vi "PT (Main).vi"(7 "Name of Parent Panel":string="Main.vi", 9 "New Center Coords":T1={"Horizontal"=470, "Vertical"=200}, 10 "Config":variant, 11 "Main UI Message Queue":refnum<queue>) -> ()   [LabVIEW 2018, in "PT Module.lvlib"]
doc: "This Continuous Measurement sample project is based on the Queued Message Handler template.\n\nThe Event Handling Loop generates messages based on user interface actions.\n\nThe Message Handling Loop processes messages generated by the Event Handling Loop, or by other messages. There are also Acquisition and Logging message handling loop subVIs, and a chart updating loop."
uses:
  PT Module.lvlib
  support/Message Queue/Message Cluster.ctl
  <vilib>/Utility/miscctls.llb/LVPoint32TypeDef.ctl
  Controls/PT Module Config Cluster.ctl
  Tag VIs/Numeric Alarm Settings Cluster.ctl
  Tag VIs/Tag FGV Operation Enum.ctl
  support/Message Queue/Enqueue Message (Single).vi
  support/User Event - Stop/User Event - Stop.lvlib
  support/Support Library.lvlib
  support/Message Queue/Message Queue.lvlib
  Shared Variables/Dynamic Shared Variables.lvlib
  subVIs/PT Settings Dialog.vi
  support/Command Log VIs/Command Logging.lvlib
panel:
  out "Numeric":dbl format="%.1f"
  out "data string 2":string
  out "data string":string
  out "xml string":string
  in  "Settings":bool
  out "Tag Name":string
  out "Input Channel Tag Name":string
  out "Pressure":dbl caption="PSIG" format="%.1f"
  in  "Start":bool
  out "Log File path":path
  in  "Force Trigger":bool
  in  "Stop":bool
  out "Status":string
  in  "Exit":bool
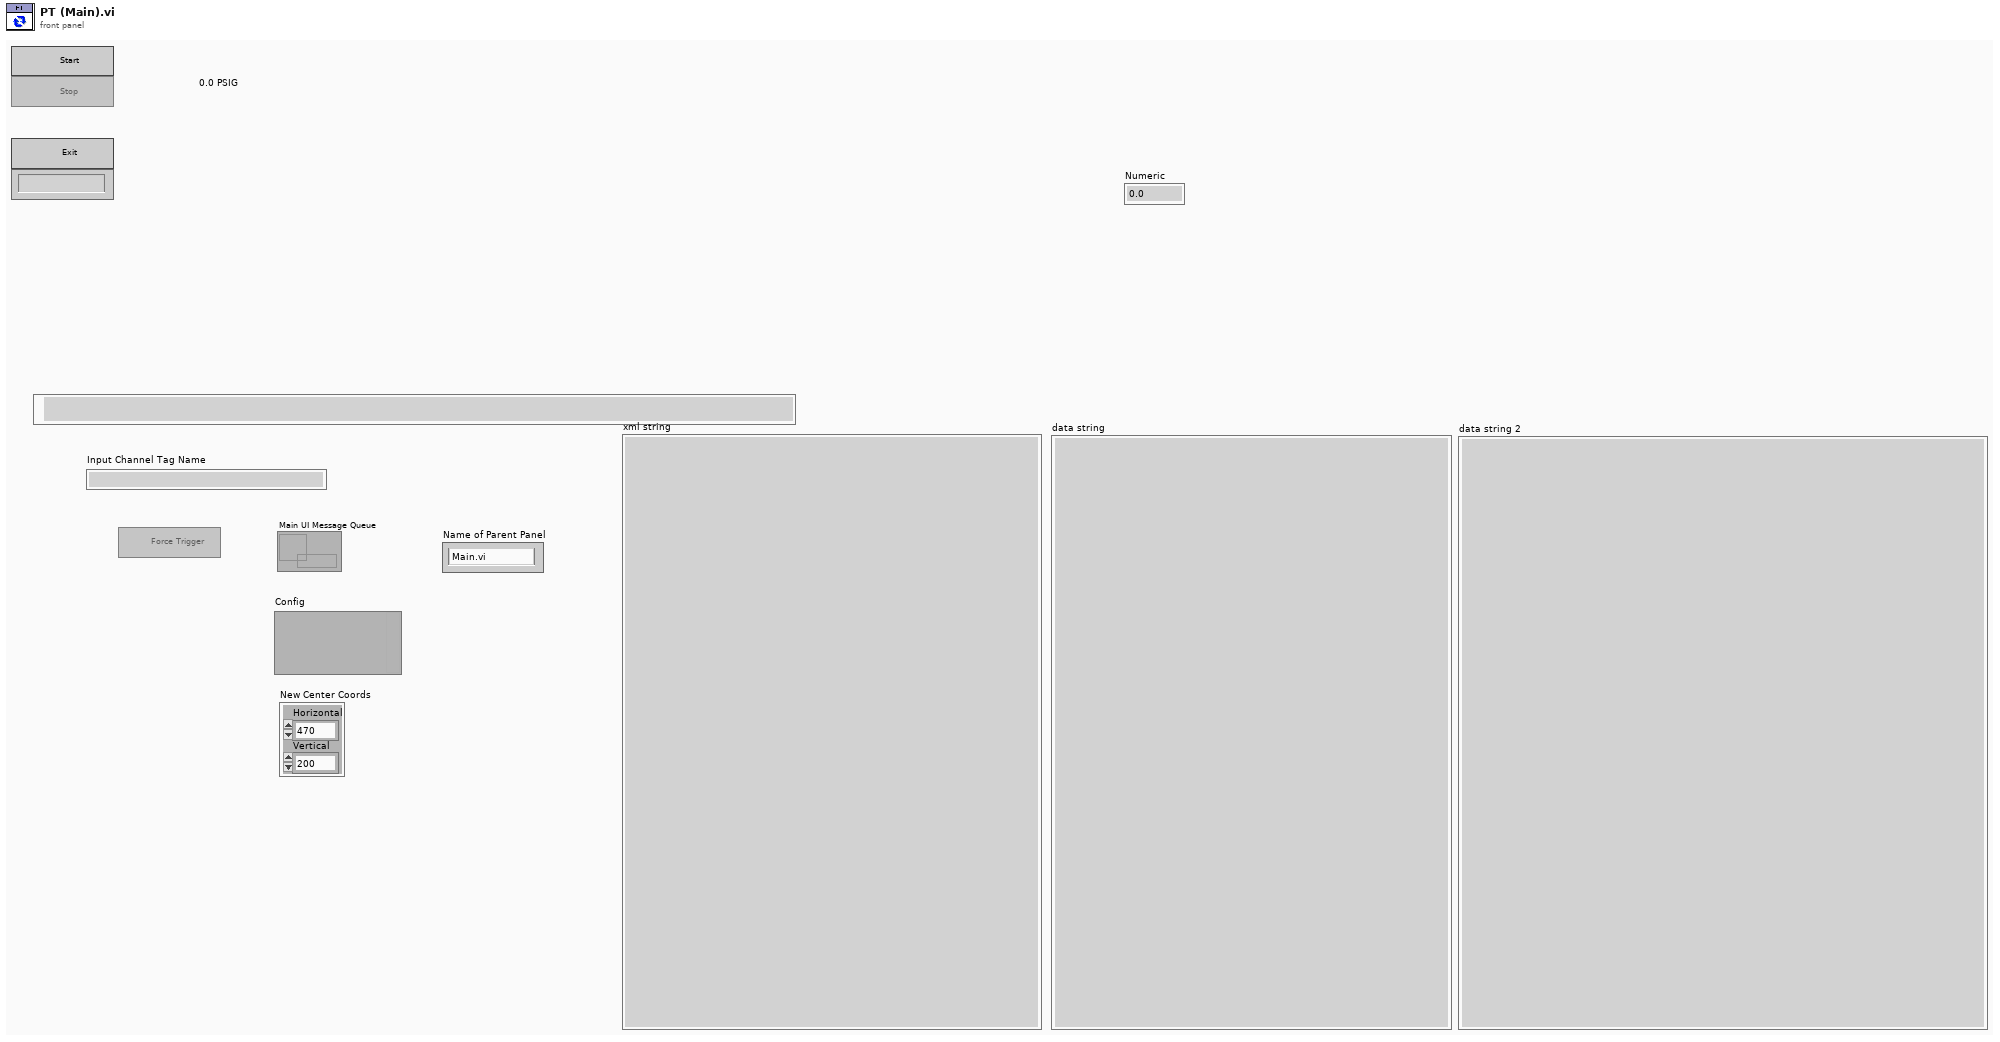
[diagram p1: front panel]
types:
  T1 = typedef "LVPoint32TypeDef.ctl" = cluster{"Horizontal":i32, "Vertical":i32}
  T2 = typedef "PT Module.lvlib/PT Module Config Cluster.ctl" = cluster{"GUID":string, "Drop Coords":T1, "Input Channel Tag Name ":string, "Process Name":string, "Queue Name":string, "Input Channel Numeric Alarm Settings":T3[]}
  T3 = typedef "Numeric Alarm Settings Cluster.ctl" = cluster{"enable? (F)":bool, "name":string, "alarm type":enum16{"HI_HI", "HI", "LO", "LO_LO"}, "level/change":dbl, "deadband/time":dbl, "alarm delay":dbl, "priority":u32, "ack type":enum16{"Auto", "User", "None", "Each Occurrence"}, "area":string, "description":string, "log? (T)":bool}
  T4 = typedef "Tag FGV Operation Enum.ctl" = enum16{"Init", "Set Notification Queue", "Create Tag", "Commit", "Write Tag (Numeric)", "Write Tag (Boolean)", "Read All Tags", "Read One Tag", "Delete Tag Category", "Set Alarm Parameters (Numeric)", "Set Alarm Parameters (Boolean)", "Enable All Alarms", "Disable All Alarms", "Delete All Tags", "Read Alarms", "Ack Alarm", "Read Alarm Parameters (Numeric)", "Read Alarm Parameters (Boolean)"}
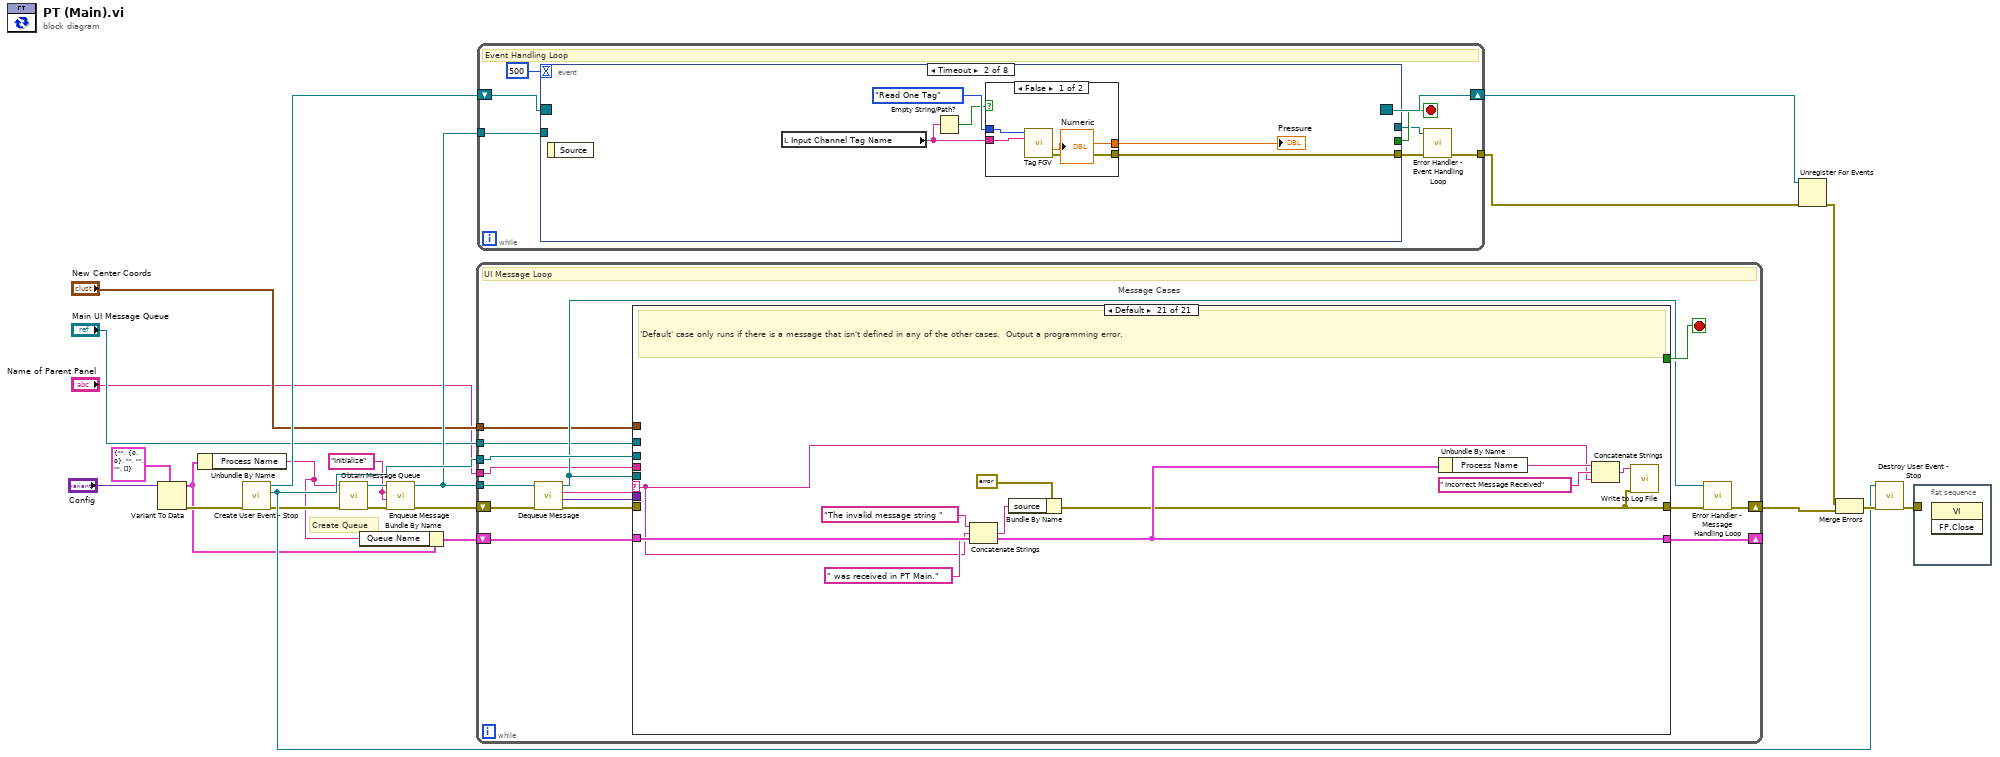
[diagram p0: block diagram]
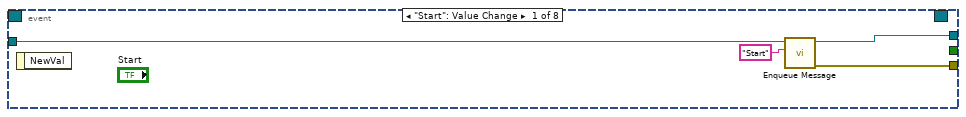
[diagram p2: hidden frame]
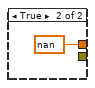
[diagram p3: hidden frame]
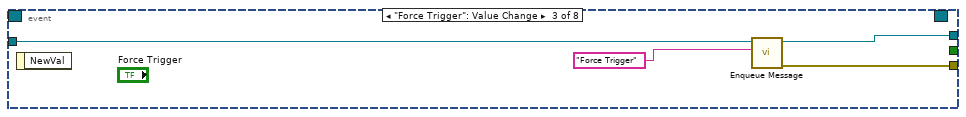
[diagram p4: hidden frame]
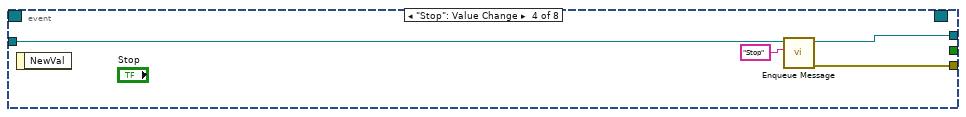
[diagram p5: hidden frame]
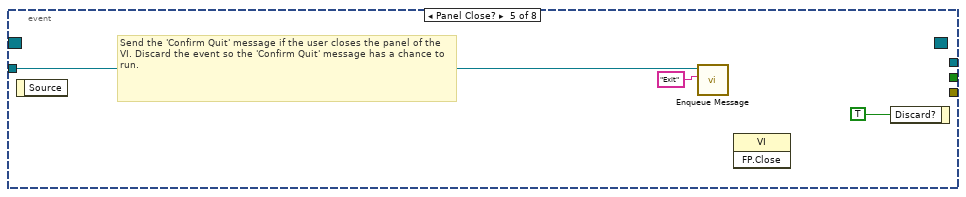
[diagram p6: hidden frame]
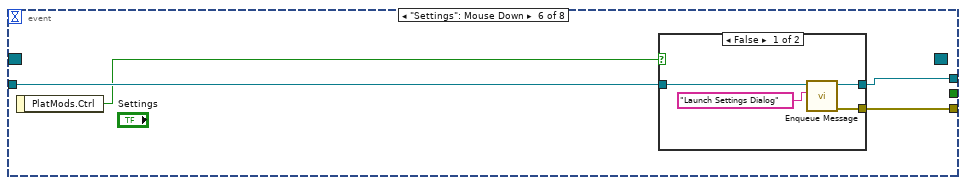
[diagram p7: hidden frame]
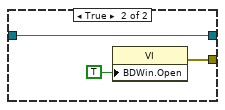
[diagram p8: hidden frame]
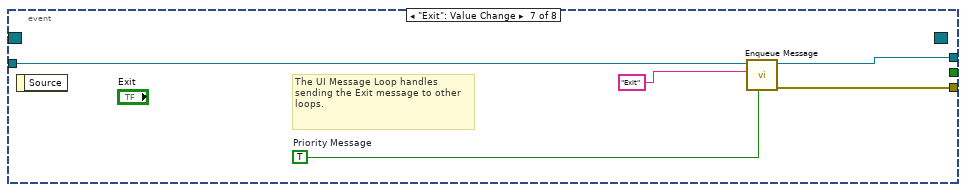
[diagram p9: hidden frame]
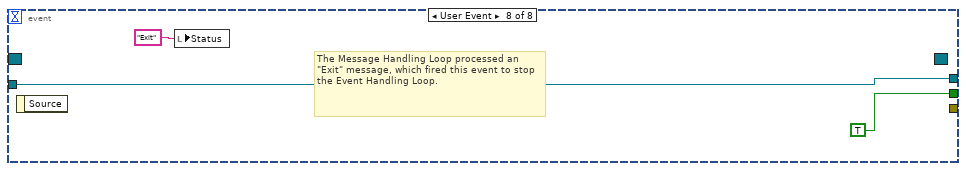
[diagram p10: hidden frame]
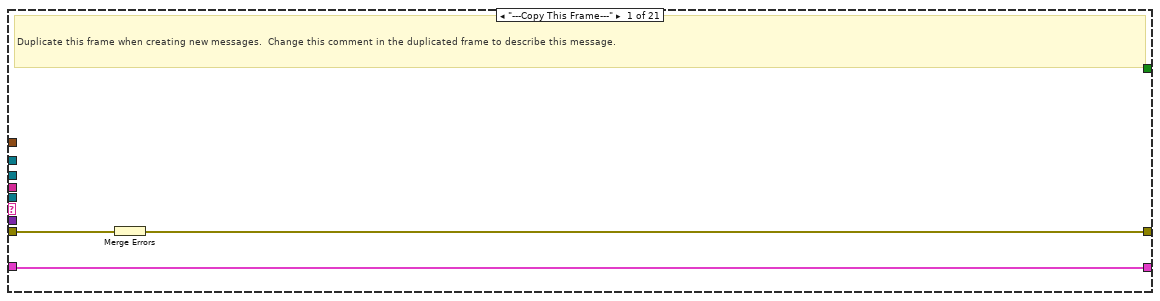
[diagram p11: hidden frame]
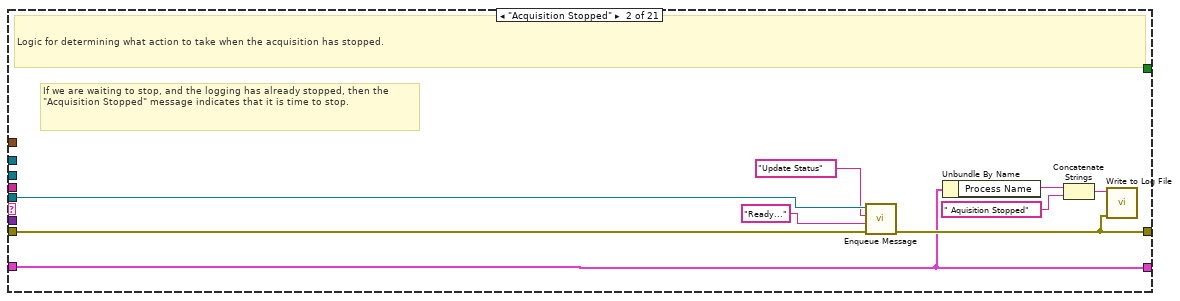
[diagram p12: hidden frame]
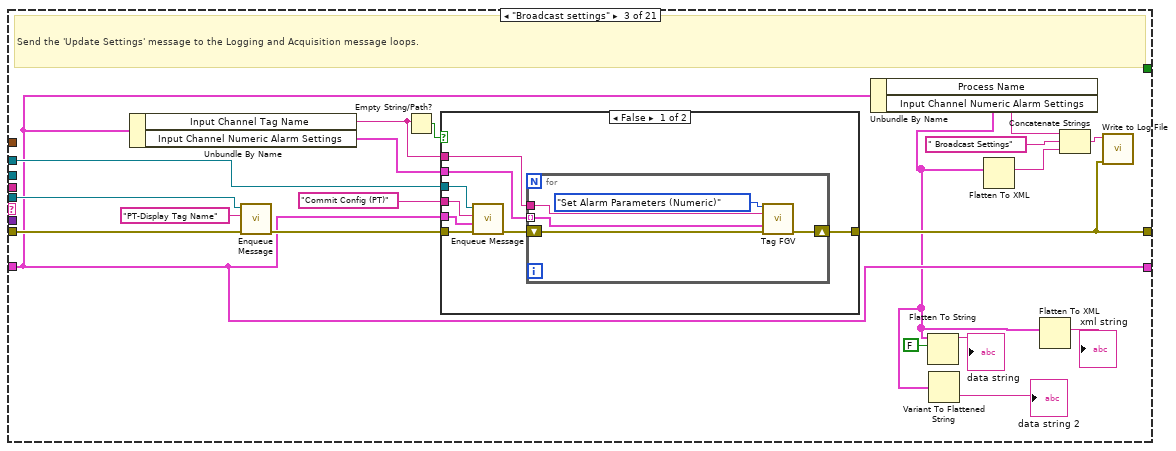
[diagram p13: hidden frame]
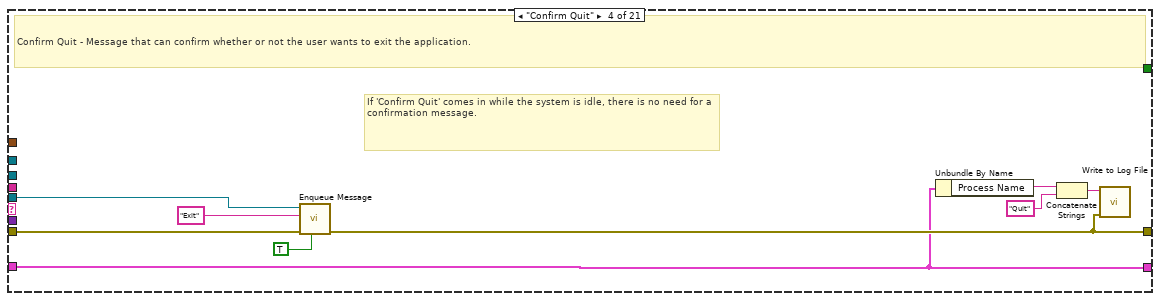
[diagram p15: hidden frame]
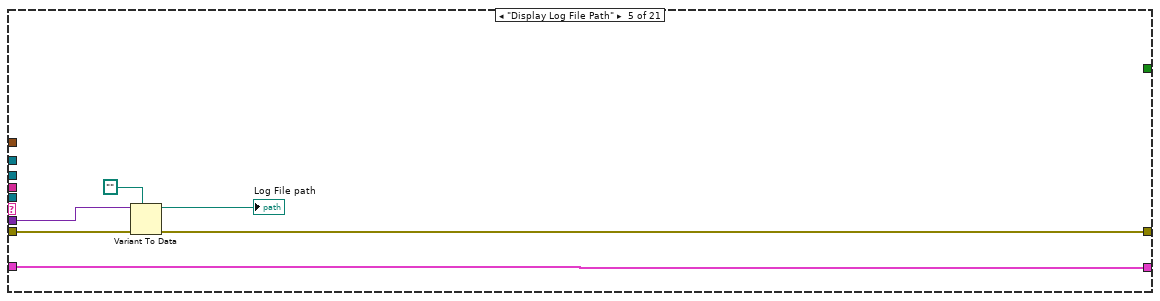
[diagram p16: hidden frame]
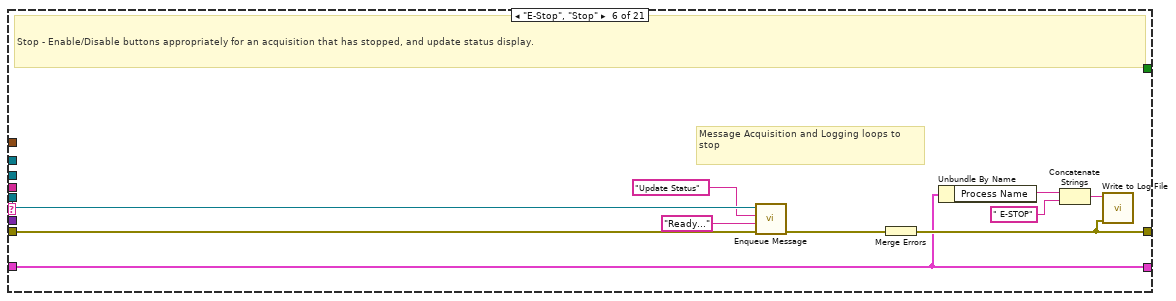
[diagram p17: hidden frame]
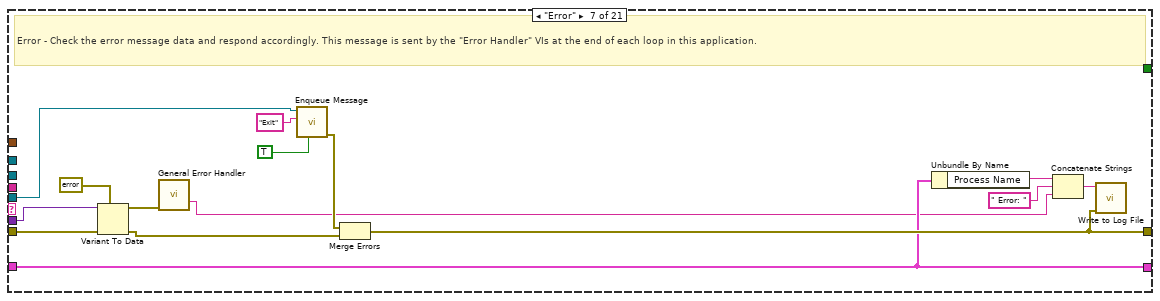
[diagram p18: hidden frame]
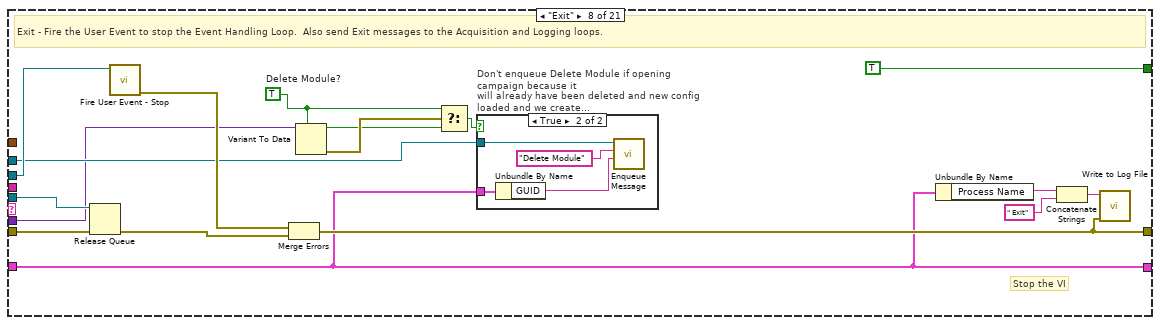
[diagram p19: hidden frame]
diagram:
  w13 = "Initialize" ("Message")
  # "Create Queue"
  n1 = Variant To Data(type=T2 {"GUID"="", "Drop Coords"={"Horizontal"=0, "Vertical"=0}, "Input Channel Tag Name "="", "Process Name"="", "Queue Name"="", "Input Channel Numeric Alarm Settings"=[]} ("TT Module Config"), Variant="Config") -> (data=w2:T2, error out=w7:errorcluster)  [unwired: 1 in]
  n2 = Unbundle By Name(w2) -> ("Process Name"=w3:string)
  n3 = call "Create User Event - Stop.vi"("error in (no error)"=w7) -> ("error out"=w11:errorcluster, "User Event - Stop"=w19:refnum<user-event>, "Stop Event Registration Refnum"=w20:refnum<event-registration>)  [unwired: 8 in]
  n4 = call "Obtain Message Queue.vi"("error in (no error)"=w11, "name (unnamed)"=w3) -> ("error out"=w16:errorcluster, "Message Queue"=w15:refnum<queue>)  [unwired: 8 in]
  n5 = Bundle By Name(cluster=w2, "Queue Name"=w3) -> (w1:T2)
  n6 = call-poly "Enqueue Message.vi"("error in (no error)"=w16, "Message Data"=w13, "Message"=w13, "Message Queue"=w15) -> ("error out"=w12:errorcluster, "dup Message Queue"=w14:refnum<queue>)  [unwired: 6 in]
  n7 = while {
    tunnel: w14 -> [w32]
    tunnel: w19 -> [w37]
    shift-right: [w28] -> w23
    shift-left: w12 -> [w36]
    shift-right: [w31] -> _
    shift-left: w1 -> [w30]
    tunnel: "Main UI Message Queue" -> [w26]
    tunnel: "New Center Coords" -> [w25]
    tunnel: "Name of Parent Panel" -> [w24]
    stop <- w38 stop-if-true
    # "UI Message Loop"
    n8 = call "Dequeue Message.vi"("error in (no error)"=w36, "Message Queue"=w32) -> ("error out"=w35:errorcluster, "Message Data"=w33:variant, "Message"=w34:string, "dup Message Queue"=w27:refnum<queue>)  [unwired: 6 in]
    n9 = case "Message Cases" shown="Default" w34 {
      selector: w34 -> [_ _ _ _ _ _ _ _ _ _ _ _ _ _ _ _ _ _ _ _ w248]
      tunnel: w27 -> [_ w49 w68 w93 _ w109 w120 w137 _ _ w174 w184 _ _ w201 w206 w225 _ _ _ _]
      tunnel: w35 -> [w41 w50 w70 w92 w94 w106 w124 w140 w146 w159 w171 w188 w194 w196 w200 w207 w223 w230 w237 w245 _]
      tunnel: [w40 w43 w58 w86 w95 w101 w112 w126 w148 w159 w160 w180 w194 w196 w199 w205 w219 w230 w236 w246 w247] -> w29
      tunnel: [_ _ _ _ _ _ _ TRUE _ _ _ _ _ _ _ _ _ _ _ _ _] -> w38
      tunnel: w33 -> [_ _ _ _ w97 _ w123 w130 _ _ _ _ _ _ _ _ _ _ _ w244 _]
      tunnel: w37 -> [_ _ _ _ _ _ _ w139 _ _ _ _ _ _ _ _ _ _ _ _ _]
      tunnel: [w39 w42 w57 w85 w99 w100 w111 w125 w147 w158 w161 w179 w195 w197 w204 w210 w218 w231 w232 w241 w253] -> w31
      tunnel: w30 -> [w39 w42 w57 w85 w99 w100 w111 w125 w147 w158 w161 w185 w195 w197 w204 w210 w218 w231 w232 w241 w253]
      tunnel: w26 -> [_ _ w69 _ _ _ _ w131 _ _ _ _ _ _ _ _ _ _ w238 _ _]
      tunnel: w25 -> [_ _ _ _ _ _ _ _ _ _ w167 _ _ _ _ _ _ _ _ _ _]
      tunnel: w24 -> [_ _ _ _ _ _ _ _ _ _ w166 _ _ _ _ _ _ _ _ _ _]
      frame "---Copy This Frame---" {
        # "Duplicate this frame when creating new messages.  Change this comment in the duplicated frame to describe this message."
        n10 = Merge Errors(w41) -> (w40:errorcluster)
      }
      frame "Acquisition Stopped" {
        # "If we are waiting to stop, and the logging has already stopped, then the \"Acquisition Stopped\" message indicates that it is time to stop."
        # "Logic for determining what action to take when the acquisition has stopped."
        n11 = call-poly "Enqueue Message.vi"("error in (no error)"=w50, "Message Data"="Ready..." ("Message"), "Message"="Update Status", "Message Queue"=w49) -> ("error out"=w43:errorcluster)  [unwired: 6 in, 1 out]
        n12 = Unbundle By Name(w42) -> ("Process Name"=w46:string)
        n13 = Concatenate Strings(w46, " Aquisition Stopped" ("text")) -> (w45:string)
        n14 = call "Write to Log File.vi"("error in"=w43, "text"=w45) -> ()  [unwired: 9 in, 1 out]
      }
      frame "Broadcast settings" {
        # "Send the 'Update Settings' message to the Logging and Acquisition message loops."
        n15 = Unbundle By Name(w57) -> ("Input Channel Tag Name"=w62:string, "Input Channel Numeric Alarm Settings"=w66:T3[])
        n16 = call-poly "Enqueue Message.vi"("error in (no error)"=w70, "Message"="PT-Display Tag Name", "Message Queue"=w68) -> ("error out"=w64:errorcluster)  [unwired: 7 in, 1 out]
        n17 = Empty String/Path?(string/path=w62) -> (empty?=w65:bool)
        n18 = case shown="False" w65 {
          tunnel: w66 -> [w78 _]
          tunnel: [w77 w84] -> w58
          tunnel: w64 -> [w76 w84]
          tunnel: w57 -> [w75 _]
          tunnel: "Commit Config (PT)" ("Message") -> [w74 _]
          tunnel: w69 -> [w73 _]
          tunnel: w62 -> [w71 _]
          frame False {
            n19 = call-poly "Enqueue Message.vi"("error in (no error)"=w76, "Message Data"=w75, "Message"=w74, "Message Queue"=w73) -> ("error out"=w72:errorcluster)  [unwired: 6 in, 1 out]
            n20 = for {
              tunnel: w78 -> [w82] mode=indexing
              tunnel: w71 -> [w81]
              shift-right: [w79] -> w77
              shift-left: w72 -> [w80]
              n21 = call "Tag FGV.vi"("Operation"=Tag_FGV_Operation_Enum."Set Alarm Parameters (Numeric)", "Tag Name"=w81, "Data"=w82, "error in (no error)"=w80) -> ("error out"=w79:errorcluster)  [unwired: 4 in, 7 out]
            }
          }
          frame True {
          }
        }
        n22 = Unbundle By Name(w57) -> ("Process Name"=w61:string, "Input Channel Numeric Alarm Settings"=w51:T3[])
        n23 = Flatten To String(anything=w51, prepend array or string size? (T)=FALSE) -> (data string=→"data string":string)  [unwired: 2 in, 2 out]
        n24 = Variant To Flattened String(Variant=w51) -> (data string=→"data string 2":string)  [unwired: 1 out]
        n25 = Flatten To XML(anything=w51) -> (xml string=w56:string)
        n26 = Flatten To XML(anything=w51) -> (xml string=→"xml string":string)
        n27 = Concatenate Strings(w61, " Broadcast Settings" ("text"), w56) -> (w60:string)
        n28 = call "Write to Log File.vi"("error in"=w58, "text"=w60) -> ()  [unwired: 9 in, 1 out]
      }
      frame "Confirm Quit" {
        # "If 'Confirm Quit' comes in while the system is idle, there is no need for a confirmation message."
        # "Confirm Quit - Message that can confirm whether or not the user wants to exit the application."
        n29 = call-poly "Enqueue Message.vi"("Priority Message? (F)"=TRUE, "error in (no error)"=w92, "Message"="Exit", "Message Queue"=w93) -> ("error out"=w86:errorcluster)  [unwired: 6 in, 1 out]
        n30 = Unbundle By Name(w85) -> ("Process Name"=w89:string)
        n31 = Concatenate Strings(w89, "Quit" ("text")) -> (w88:string)
        n32 = call "Write to Log File.vi"("error in"=w86, "text"=w88) -> ()  [unwired: 9 in, 1 out]
      }
      frame "Display Log File Path" {
        n33 = Variant To Data(error in=w94, type=path "", Variant=w97) -> (data=→"Log File path":path, error out=w95:errorcluster)
      }
      frame "E-Stop", "Stop" {
        # "Message Acquisition and Logging loops to stop"
        # "Stop - Enable/Disable buttons appropriately for an acquisition that has stopped, and update status display."
        n34 = call-poly "Enqueue Message.vi"("error in (no error)"=w106, "Message Data"="Ready..." ("Ready..."), "Message"="Update Status", "Message Queue"=w109) -> ("error out"=w105:errorcluster)  [unwired: 6 in, 1 out]
        n35 = Merge Errors(w105) -> (w101:errorcluster)
        n36 = Unbundle By Name(w100) -> ("Process Name"=w104:string)
        n37 = Concatenate Strings(w104, " E-STOP" ("text")) -> (w103:string)
        n38 = call "Write to Log File.vi"("error in"=w101, "text"=w103) -> ()  [unwired: 9 in, 1 out]
      }
      frame "Error" {
        # "Error - Check the error message data and respond accordingly. This message is sent by the \"Error Handler\" VIs at the end of each loop in this application."
        n39 = Variant To Data(error in=w124, type=errorcluster {"status"=FALSE, "code"=0, "source"=""} ("error out"), Variant=w123) -> (data=w121:errorcluster, error out=w117:errorcluster)
        n40 = call <vilib>:"General Error Handler.vi"("error in (no error)"=w121) -> ("message"=w110:string)  [unwired: 10 in, 4 out]
        n41 = call-poly "Enqueue Message.vi"("Priority Message? (F)"=TRUE, "Message"="Exit", "Message Queue"=w120) -> ("error out"=w116:errorcluster)  [unwired: 7 in, 1 out]
        n42 = Merge Errors(w116, w117) -> (w112:errorcluster)
        n43 = Unbundle By Name(w111) -> ("Process Name"=w115:string)
        n44 = Concatenate Strings(w115, " Error: " ("text"), w110) -> (w114:string)
        n45 = call "Write to Log File.vi"("error in"=w112, "text"=w114) -> ()  [unwired: 9 in, 1 out]
      }
      frame "Exit" {
        w134 = TRUE  # Delete Module?
        # "Stop the VI"
        # "Exit - Fire the User Event to stop the Event Handling Loop.  Also send Exit messages to the Acquisition and Logging loops."
        n46 = Release Queue(queue=w137, error in (no error)=w140) -> (error out=w136:errorcluster)  [unwired: 1 in, 2 out]
        n47 = call "Fire User Event - Stop.vi"("User Event - Stop"=w139) -> ("error out"=w138:errorcluster)  [unwired: 10 in]
        n48 = Merge Errors(w138, w136) -> (w126:errorcluster)
        n49 = Variant To Data(type=w134, Variant=w130) -> (data=w133:bool, error out=w135:errorcluster)  [unwired: 1 in]
        n50 = Select(t=w134, s=w135, f=w133) -> (s? t:f=w132:bool)
        n51 = case "Don't enqueue Delete Module if opening campaign because it\nwill already have been deleted and new config loaded and we create\na race condition." shown="True" w132 {
          tunnel: w131 -> [_ w144]
          tunnel: w125 -> [_ w143]
          frame False {
          }
          frame True {
            n52 = Unbundle By Name(w143) -> ("GUID"=w142:string)
            n53 = call-poly "Enqueue Message.vi"("Message Data"=w142, "Message"="Delete Module", "Message Queue"=w144) -> ()  [unwired: 7 in, 2 out]
          }
        }
        n54 = Unbundle By Name(w125) -> ("Process Name"=w129:string)
        n55 = Concatenate Strings(w129, " Exit" ("text")) -> (w128:string)
        n56 = call "Write to Log File.vi"("error in"=w126, "text"=w128) -> ()  [unwired: 9 in, 1 out]
      }
      frame "Force Trigger" {
        # "Force Trigger - send a message to the Logging message loop to start logging."
        n57 = Merge Errors(w146) -> (w148:errorcluster)
      }
      frame "Init UI Refs" {
        # "Init UI Refs - Store control references for UI controls.  Also enable/disable controls appropriately."
        n58 = control-ref of="Status"() -> ()  [unwired: 1 out]
        n59 = property class="VI"("Front Panel.Closeable"=TRUE ("Front Panel Window:Closeable")) -> ()  [unwired: 2 in, 2 out]
        n60 = control-ref of="Force Trigger"() -> (w151:refnum<vi>)
        n61 = control-ref of="Stop"() -> (w150:refnum<vi>)
        n62 = control-ref of="Exit"() -> (w152:refnum<vi>)
        n63 = control-ref of="Start"() -> (w155:refnum<vi>)
        n64 = Build Array(w150, w151) -> (w149:refnum<vi>[])
        n65 = Build Array(w152, w155) -> (w154:refnum<vi>[])
        n66 = call "Set Enable State on Multiple Controls.vi"("Enable?"=FALSE, "Controls"=w149) -> ()  [unwired: 10 in]
        n67 = call "Set Enable State on Multiple Controls.vi"("Enable?"=TRUE, "Controls"=w154) -> ()  [unwired: 10 in]
      }
      frame "Initialize" {
        # "Initialize - Get configuration settings, then message the UI to initialize, and broadcast the settings to the other message loops."
        n68 = Unbundle By Name(w161) -> ("Process Name"=w165:string)
        n69 = property class="VI"("Front Panel.Title"=w165) -> ()  [unwired: 2 in, 2 out]
        n70 = property class="VI" props=["FP.State"]() -> (reference out=w168:refnum<vi>)  [unwired: 2 in, 2 out]
        n71 = call "Make Child and Move.vi"("Process Name"=w165, "Name of Parent Panel"=w166, "New Center Coords"=w167, "VI in"=w168) -> ()  [unwired: 8 in]
        n72 = call-poly "Enqueue Message.vi"("error in (no error)"=w171, "Message"="Init UI Refs", "Message Queue"=w174) -> ("error out"=w172:errorcluster, "dup Message Queue"=w173:refnum<queue>)  [unwired: 7 in]
        n73 = call-poly "Enqueue Message.vi"("error in (no error)"=w172, "Message"="Broadcast Settings", "Message Queue"=w173) -> ("error out"=w169:errorcluster, "dup Message Queue"=w170:refnum<queue>)  [unwired: 7 in]
        n74 = call-poly "Enqueue Message.vi"("error in (no error)"=w169, "Message Data"="Ready..." ("Ready..."), "Message"="Update Status", "Message Queue"=w170) -> ("error out"=w160:errorcluster)  [unwired: 6 in, 1 out]
        n75 = Unbundle By Name(w161) -> ("Process Name"=w164:string)
        n76 = Concatenate Strings(w164, " Initialize" ("text")) -> (w163:string)
        n77 = call "Write to Log File.vi"("error in"=w160, "text"=w163) -> ()  [unwired: 9 in, 1 out]
      }
      frame "Launch Settings Dialog" {
        # "Launch the Settings Dialog when the user clicks the 'Settings' button."
        n78 = call-by-ref "?"("error in (no error)"=w188, "PT Module Config in"=w185) -> ("error out"=w186:errorcluster, "Cancelled?"=w187:bool, "PT Module Config out"=w179:T2)  [unwired: 8 in, 3 out]
        n79 = case shown="False" w187 {
          tunnel: w186 -> [w190 w193]
          tunnel: [w192 w193] -> w180
          tunnel: w179 -> [_ _]
          tunnel: w184 -> [w189 _]
          frame False {
            n80 = call-poly "Enqueue Message.vi"("error in (no error)"=w190, "Message"="Broadcast settings", "Message Queue"=w189) -> ("error out"=w192:errorcluster)  [unwired: 7 in, 1 out]
          }
          frame True {
          }
        }
        n81 = Unbundle By Name(w179) -> ("Process Name"=w183:string)
        n82 = Concatenate Strings(w183, " Settings Dialog Launched" ("text")) -> (w182:string)
        n83 = call "Write to Log File.vi"("error in"=w180, "text"=w182) -> ()  [unwired: 9 in, 1 out]
      }
      frame "Logging Stopped" {
        # "Logic for determining what action to take when the logging has stopped."
      }
      frame "PT-Display Tag Name" {
        n84 = Unbundle By Name(w197) -> ("Input Channel Tag Name"=→"Input Channel Tag Name" →"Tag Name":string)
      }
      frame "Send to Sequence" {
        n85 = local read "Pressure"() -> (w203:dbl)
        n86 = call-poly "Enqueue Message.vi"("error in (no error)"=w200, "Message Data"=w203, "Message"="Sent to Sequence", "Message Queue"=w201) -> ("error out"=w199:errorcluster)  [unwired: 6 in, 1 out]
      }
      frame "Sent to Sequence" {
        n87 = local read "Pressure"() -> (w208:dbl)
        n88 = flat-sequence {
          tunnel: w207 -> [w215]
          tunnel: w206 -> [w213]
          tunnel: [w214] -> w209
          tunnel: w208 -> [w211]
          tunnel: [w217] -> w205
          tunnel: w209 -> [w217]
          frame #0 {
            n89 = call-poly "Enqueue Message.vi"("error in (no error)"=w215, "Message Data"=w211, "Message"="Sent to Sequence", "Message Queue"=w213) -> ("error out"=w214:errorcluster)  [unwired: 6 in, 1 out]
          }
          frame #1 {
            n90 = Wait (ms)(milliseconds to wait=u32 50) -> ()  [unwired: 1 out]
          }
        }
      }
      frame "Start" {
        # "Message Acquisition and Logging loops to start"
        # "Start - Enable/Disable buttons appropriately for an acquisition that has started, and update status display."
        n91 = call-poly "Enqueue Message.vi"("error in (no error)"=w223, "Message"="Broadcast settings", "Message Queue"=w225) -> ("error out"=w226:errorcluster, "dup Message Queue"=w224:refnum<queue>)  [unwired: 7 in]
        n92 = call-poly "Enqueue Message.vi"("error in (no error)"=w226, "Message"="Start Loops", "Message Queue"=w224) -> ("error out"=w227:errorcluster)  [unwired: 7 in, 1 out]
        n93 = Merge Errors(w227) -> (w219:errorcluster)
        n94 = Unbundle By Name(w218) -> ("Process Name"=w222:string)
        n95 = Concatenate Strings(w222, " Start" ("text")) -> (w221:string)
        n96 = call "Write to Log File.vi"("error in"=w219, "text"=w221) -> ()  [unwired: 9 in, 1 out]
      }
      frame "Start Loops" {
        # "Message Acquisition and Logging loops to start"
        # "Start - Enable/Disable buttons appropriately for an acquisition that has started, and update status display."
      }
      frame "Start Log" {
        # "The Tags are created in the DAQ Loop, but we need the \"Tags Created\" message count to = the # of modules dropped."
        n97 = call-poly "Enqueue Message.vi"("error in (no error)"=w237, "Message"="Tags Created", "Message Queue"=w238) -> ("error out"=w236:errorcluster)  [unwired: 7 in, 1 out]
        n98 = Unbundle By Name(w232) -> ("Process Name"=w235:string)
        n99 = Concatenate Strings(w235, " Tags Made" ("text")) -> (w234:string)
        n100 = call "Write to Log File.vi"("text"=w234) -> ()  [unwired: 10 in, 1 out]
      }
      frame "Update Status" {
        # "Update Display - Convert the message data to a string to display in the Status indicator."
        n101 = Variant To Data(error in=w245, type="", Variant=w244) -> (data=→"Status":string, error out=w242:errorcluster)
        n102 = Merge Errors(w242) -> (w246:errorcluster)
      }
      frame Default {
        # "'Default' case only runs if there is a message that isn't defined in any of the other cases.  Output a programming error."
        n103 = Concatenate Strings("The invalid message string " ("string"), w248, " was received in PT Main." ("string")) -> (w249:string)
        n104 = Bundle By Name(cluster=errorcluster {"status"=TRUE, "code"=1, "source"=""} ("error constant"), "source"=w249) -> (w247:errorcluster)
        n105 = Unbundle By Name(w253) -> ("Process Name"=w256:string)
        n106 = Concatenate Strings(w256, " Incorrect Message Received" ("text"), w248) -> (w255:string)
        n107 = call "Write to Log File.vi"("error in"=w247, "text"=w255) -> ()  [unwired: 9 in, 1 out]
      }
    }
    n108 = call "Error Handler - Message Handling Loop.vi"("error in (no error)"=w29, "Message Queue"=w27) -> ("dup error in"=w28:errorcluster)  [unwired: 8 in, 1 out]
  }
  n109 = while {
    tunnel: w14 -> [w263]
    tunnel: [w258] -> w22
    shift-right: [w262] -> w17
    shift-left: w20 -> [w264]
    stop <- w261 stop-if-true
    # "Event Handling Loop"
    n110 = event shown="[1] Timeout" {
      selector: w264 -> [_ _ _ _ _ _ _ _]
      dyn-events: [_ _ _ _ _ _ _ _] -> w262
      timeout: 500 -> [_ _ _ _ _ _ _ _]
      tunnel: [_ _ _ _ _ _ _ TRUE ("Discard?")] -> w261
      tunnel: w263 -> [w266 _ w281 w285 w287 w292 w302 w306]
      tunnel: [w268 w271 w280 w284 _ w293 w305 _] -> w259
      tunnel: [w265 _ w279 w283 _ w291 w301 w306] -> w260
      event "Start": Value Change {
        n111 = event-data() -> ()  [unwired: 1 in, 1 out]
        n112 = call-poly "Enqueue Message.vi"("Message"="Start", "Message Queue"=w266) -> ("error out"=w268:errorcluster, "dup Message Queue"=w265:refnum<queue>)  [unwired: 8 in]
      }
      event Timeout {
        n113 = event-data() -> ()  [unwired: 1 in, 1 out]
        n114 = local read "Input Channel Tag Name"() -> (w270:string)
        n115 = Empty String/Path?(string/path=w270) -> (empty?=w269:bool)
        n116 = case shown="False" w269 {
          tunnel: Tag_FGV_Operation_Enum."Read One Tag" ("Operation") -> [w277 _]
          tunnel: [w276 nan ("Tag Value")] -> w272
          tunnel: [w275 _] -> w271
          tunnel: w270 -> [w274 _]
          frame False {
            n117 = call "Tag FGV.vi"("Operation"=w277, "Tag Name"=w274) -> ("Tag Value"=w276:dbl, "error out"=w275:errorcluster)  [unwired: 6 in, 6 out]
          }
          frame True {
          }
        }
        "Pressure" <- w272
      }
      event "Force Trigger": Value Change {
        n118 = event-data() -> ()  [unwired: 1 in, 1 out]
        n119 = call-poly "Enqueue Message.vi"("Message"="Force Trigger", "Message Queue"=w281) -> ("error out"=w280:errorcluster, "dup Message Queue"=w279:refnum<queue>)  [unwired: 8 in]
      }
      event "Stop": Value Change {
        n120 = event-data() -> ()  [unwired: 1 in, 1 out]
        n121 = call-poly "Enqueue Message.vi"("Message"="Stop", "Message Queue"=w285) -> ("error out"=w284:errorcluster, "dup Message Queue"=w283:refnum<queue>)  [unwired: 8 in]
      }
      event Panel Close? {
        # "Send the 'Confirm Quit' message if the user closes the panel of the VI. Discard the event so the 'Confirm Quit' message has a chance to run."
        n122 = event-data() -> ()  [unwired: 1 in, 1 out]
        n123 = call-poly "Enqueue Message.vi"("Message"="Exit", "Message Queue"=w287) -> ()  [unwired: 8 in, 2 out]
        n124 = invoke class="VI" method="FP.Close"() -> ()  [unwired: 3 in, 3 out]
        n125 = event-data("Discard?"=TRUE) -> ()  [unwired: 1 in, 1 out]
      }
      event "Settings": Mouse Down {
        n126 = event-data() -> ("PlatMods.Ctrl"=w290:bool)  [unwired: 1 in]
        n127 = case shown="False" w290 {
          tunnel: [w297 w299] -> w293
          tunnel: w292 -> [w295 w298]
          tunnel: [w294 w298] -> w291
          frame False {
            n128 = call-poly "Enqueue Message.vi"("Message"="Launch Settings Dialog", "Message Queue"=w295) -> ("error out"=w297:errorcluster, "dup Message Queue"=w294:refnum<queue>)  [unwired: 8 in]
          }
          frame True {
            n129 = property class="VI"("BDWin.Open"=TRUE ("Block Diagram Window:Open")) -> (error out=w299:errorcluster)  [unwired: 2 in, 1 out]
          }
        }
      }
      event "Exit": Value Change {
        w303 = TRUE  # Priority Message
        # "The UI Message Loop handles sending the Exit message to other loops."
        n130 = event-data() -> ()  [unwired: 1 in, 1 out]
        n131 = call-poly "Enqueue Message.vi"("Priority Message? (F)"=w303, "Message"="Exit", "Message Queue"=w302) -> ("error out"=w305:errorcluster, "dup Message Queue"=w301:refnum<queue>)  [unwired: 7 in]
      }
      event User Event {
        # "The Message Handling Loop processed an \"Exit\" message, which fired this event to stop the Event Handling Loop."
        n132 = event-data() -> ()  [unwired: 1 in, 1 out]
        n133 = local write "Status"("Exit" ("Exit String")) -> ()
      }
    }
    n134 = call "Error Handler - Event Handling Loop.vi"("error in (no error)"=w259, "Message Queue"=w260) -> ("dup error in"=w258:errorcluster)  [unwired: 8 in, 1 out]
  }
  n135 = Unregister For Events(event registration refnum=w17, error in=w22) -> (error out=w18:errorcluster)
  n136 = Merge Errors(w18, w23) -> (w21:errorcluster)
  n137 = call "Destroy User Event - Stop.vi"("error in (no error)"=w21, "User Event - Stop"=w19) -> ("error out"=w4:errorcluster)  [unwired: 9 in]
  n138 = flat-sequence {
    tunnel: w4 -> [_]
    frame #0 {
      n139 = invoke class="VI" method="FP.Close"() -> ()  [unwired: 3 in, 3 out]
    }
  }
